vi "FYP_VI_MIDI_NotePress.vi"(4 "MIDI Channel":u32 max=15, 5 "Pitch Note":u32 max=127, 6 "Velocity / Volume":u32 max=127, 7 "midiOut Handle":i32) -> (0 "midiOutShortMsg Error Code":i32, 3 "midiOut handle":i32)   [LabVIEW 2013]
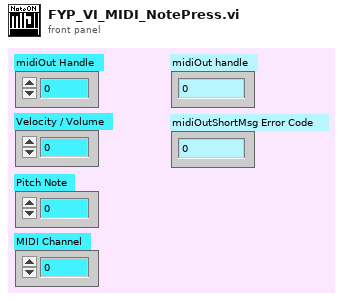
[diagram p1: front panel]
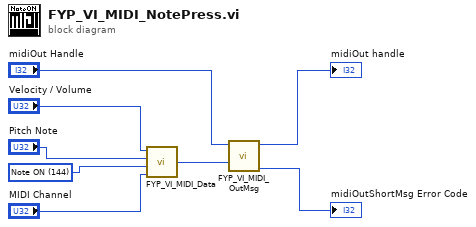
[diagram p0: block diagram]
diagram:
  w8 = u32 144 items=["Note ON"=144, "Note OFF"=128]
  n1 = call "FYP_VI_MIDI_Data.vi"("MIDI Channel"="MIDI Channel", "Mode On / Off"=w8, "Pitch Note"="Pitch Note", "Velocity / Volume"="Velocity / Volume") -> ("MIDI data"=w4:u32)
  n2 = call "FYP_VI_MIDI_OutMsg.vi"("dwMsg dataIn"=w4, "midiOut hmo"="midiOut Handle") -> ("midiOutShortMsg Error Code"=→"midiOutShortMsg Error Code":i32, "midiOut handle"=→"midiOut handle":i32)  [unwired: 4 in]
